vi "Autonomous Independent.vi"   [LabVIEW 2014]
doc: "This VI is called when autonomous begins, and will automatically be terminated when autonomous ends. You can carry out timed or sensor driven robot movement independently without needing to return to the caller."
uses:
  <vilib>/Rock Robotics/WPI/Joystick/WPI_JoystickGetSetRefNum.vi
  <vilib>/Rock Robotics/Network Tables/SD Read Number.vi
  Global 1.vi
panel:
  # "Be sure to right-click and choose Data Operations>>Make Current Value default if you want to save the array values with the VI"
types:
  T1 = typedef "WPI_JoystickDevRef.ctl" = cluster{"Device":T2}
  T2 = typedef "WPI_JoystickDeviceEnum.ctl" = enum16{"USB 0", "USB 1", "USB 2", "USB 3", "USB 4", "USB 5"}
  T3 = typedef "WPI_EncoderDevRef.ctl" = cluster{"DevStatus":errorcluster, "EncoderIndex":T4, "CounterIndex":T5, "DistancePerCount":dbl, "Decoding Type":T6}
  T4 = typedef "FPGA_EncoderIdx.ctl" = enum8{"Enc 0", "Enc 1", "Enc 2", "Enc 3", "Enc 4", "Enc 5", "Enc 6", "Enc 7", "Invalid"}
  T5 = typedef "FPGA_CounterCtrSystemIndex.ctl" = enum8{"Ctr 0", "Ctr 1", "Ctr 2", "Ctr 3", "Ctr 4", "Ctr 5", "Ctr 6", "Ctr 7", "Invalid"}
  T6 = typedef "WPI_EncoderType.ctl" = enum16{"1x", "2x", "4x"}
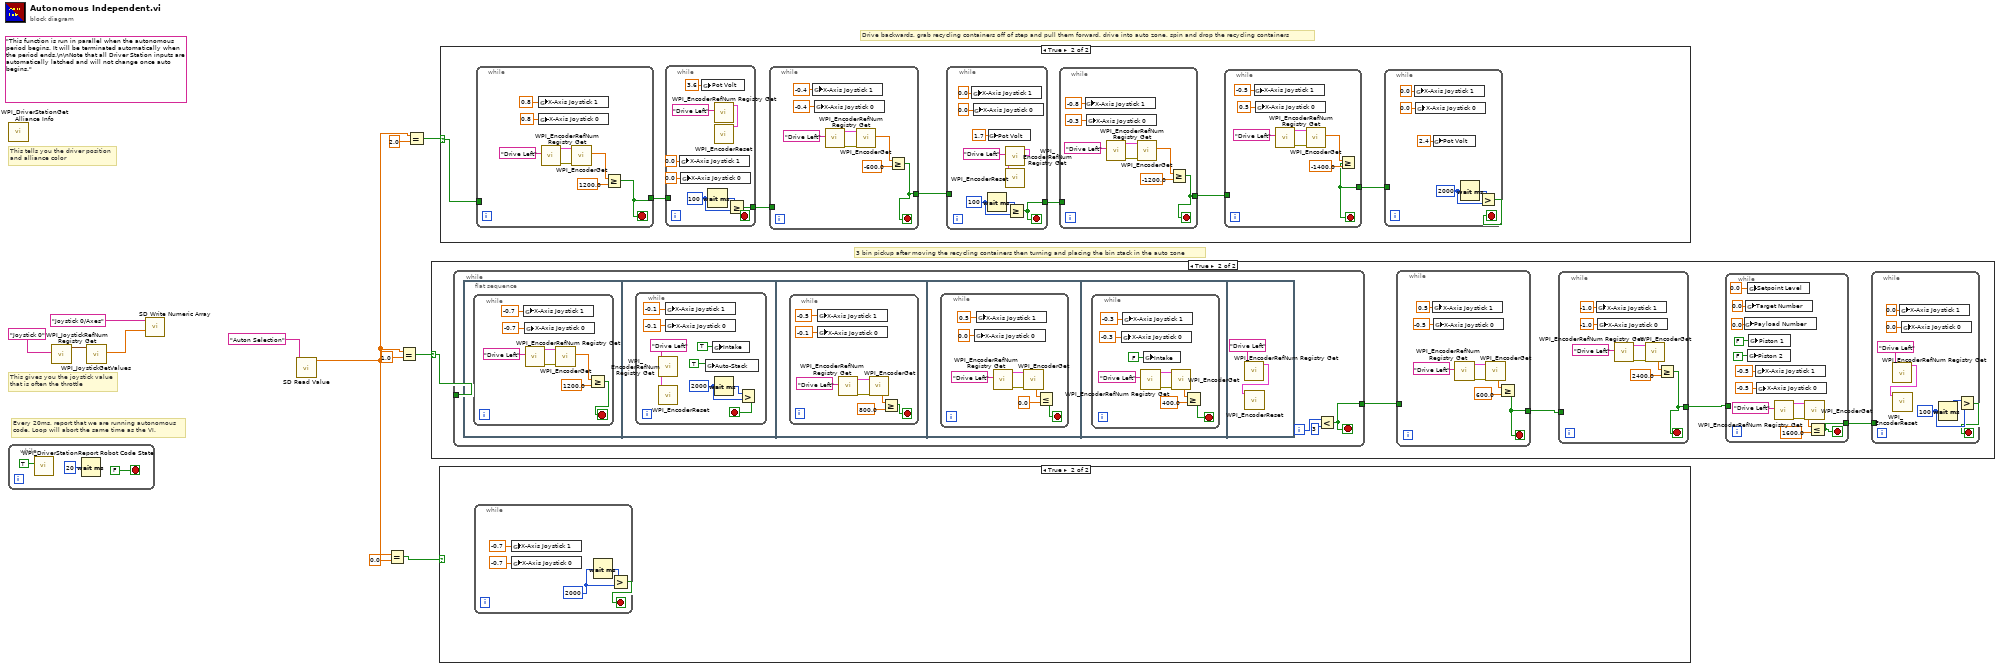
[diagram p0: block diagram]
diagram:
  (unwired) "This function is run in parallel when the autonomous period begins. It will be terminated automatically when the period ends.\n\nNote that all Driver Station inputs are automatically latched and will not change once auto begins."
  # "3 bin pickup after moving the recycling containers then turning and placing the bin stack in the auto zone"
  # "Drive backwards, grab recycling containers off of step and pull them forward, drive into auto zone, spin and drop the recycling containers"
  # "Every 20ms, report that we are running autonomous\ncode. Loop will abort the same time as the VI."
  # "This gives you the joystick value\nthat is often the throttle"
  # "This tells you the driver position\nand alliance color"
  n1 = while {
    stop <- FALSE stop-if-true
    n2 = call <vilib>:"WPI_DriverStationReport Robot Code State.vi"("Autonomous"=TRUE) -> ()  [unwired: 10 in, 1 out]
    n3 = Wait (ms)(milliseconds to wait=u32 20) -> ()  [unwired: 1 out]
  }
  n4 = call <vilib>:"WPI_DriverStationGet Alliance Info.vi"() -> ()  [unwired: 12 out]
  n5 = call <vilib>:"WPI_JoystickRefNum Registry Get.vi"("refnum name"="Joystick 0") -> ("JoystickDevRef"=w11:T1)  [unwired: 1 in, 9 out]
  n6 = call <vilib>:"WPI_JoystickGetValues.vi"("JoystickDevRef"=w11) -> ("Axes"=w9:dbl[])  [unwired: 6 in, 4 out]
  n7 = call <vilib>:"SD Write Numeric Array.vi"("Numeric Array"=w9, "Name"="Joystick 0/Axes") -> ()  [unwired: 8 in, 2 out]
  n8 = call-poly <vilib>:"SD Read Value.vi"("Name"="Auton Selection") -> ("Numeric"=w2:dbl)  [unwired: 8 in, 2 out]
  n9 = Equal?(x=w2, y=0.0) -> (x = y?=w6:bool)
  n10 = Equal?(x=w2, y=1.0) -> (x = y?=w4:bool)
  n11 = Equal?(x=w2, y=2.0) -> (x = y?=w1:bool)
  n12 = case shown="True" w4 {
    selector: w4 -> [_ w20]
    frame False {
    }
    frame True {
      n13 = while {
        tunnel: w20 -> [_]
        tunnel: [w57] -> w19
        i -> [w59]
        stop <- w57 stop-if-true
        n14 = flat-sequence {
          frame #0 {
            n15 = while {
              stop <- w60 stop-if-true
              n16 = global write "Global 1.vi" "X-Axis Joystick 1"(-0.7 ("X-Axis Joystick 1")) -> ()
              n17 = global write "Global 1.vi" "X-Axis Joystick 0"(-0.7 ("X-Axis Joystick 0")) -> ()
              n18 = call <vilib>:"WPI_EncoderRefNum Registry Get.vi"("refnum name"="Drive Left") -> ("error out"=w65:errorcluster, "EncoderDevRef"=w63:T3)  [unwired: 9 in]
              n19 = call <vilib>:"WPI_EncoderGet.vi"("error in (no error)"=w65, "EncoderDevRef"=w63) -> ("Distance"=w62:dbl)  [unwired: 4 in, 5 out]
              n20 = Greater Or Equal?(x=w62, y=1200.0) -> (x >= y?=w60:bool)
            }
          }
          frame #1 {
            n21 = while {
              stop <- w70 stop-if-true
              w71 = u32 2000 ("milliseconds to wait")
              n22 = call <vilib>:"WPI_EncoderRefNum Registry Get.vi"("refnum name"="Drive Left") -> ("EncoderDevRef"=w68:T3)  [unwired: 9 in, 1 out]
              n23 = call <vilib>:"WPI_EncoderReset.vi"("EncoderDevRef"=w68) -> ()  [unwired: 9 in, 2 out]
              n24 = global write "Global 1.vi" "X-Axis Joystick 1"(-0.1 ("X-Axis Joystick 1")) -> ()
              n25 = global write "Global 1.vi" "X-Axis Joystick 0"(-0.1 ("X-Axis Joystick 0")) -> ()
              n26 = global write "Global 1.vi" "Auto-Stack"(TRUE ("Intake")) -> ()
              n27 = global write "Global 1.vi" "Intake"(TRUE ("Intake")) -> ()
              n28 = Wait (ms)(milliseconds to wait=w71) -> (millisecond timer value=w72:u32)
              n29 = Greater?(x=w72, y=w71) -> (0:w70:bool)
            }
          }
          frame #2 {
            n30 = while {
              stop <- w77 stop-if-true
              n31 = global write "Global 1.vi" "X-Axis Joystick 1"(-0.5 ("X-Axis Joystick 1")) -> ()
              n32 = global write "Global 1.vi" "X-Axis Joystick 0"(-0.1 ("X-Axis Joystick 0")) -> ()
              n33 = call <vilib>:"WPI_EncoderRefNum Registry Get.vi"("refnum name"="Drive Left") -> ("error out"=w82:errorcluster, "EncoderDevRef"=w80:T3)  [unwired: 9 in]
              n34 = call <vilib>:"WPI_EncoderGet.vi"("error in (no error)"=w82, "EncoderDevRef"=w80) -> ("Distance"=w79:dbl)  [unwired: 4 in, 5 out]
              n35 = Greater Or Equal?(x=w79, y=800.0) -> (x >= y?=w77:bool)
            }
          }
          frame #3 {
            n36 = while {
              stop <- w85 stop-if-true
              n37 = global write "Global 1.vi" "X-Axis Joystick 0"(0.0 ("X-Axis Joystick 0")) -> ()
              n38 = global write "Global 1.vi" "X-Axis Joystick 1"(0.5 ("X-Axis Joystick 1")) -> ()
              n39 = call <vilib>:"WPI_EncoderRefNum Registry Get.vi"("refnum name"="Drive Left") -> ("error out"=w90:errorcluster, "EncoderDevRef"=w88:T3)  [unwired: 9 in]
              n40 = call <vilib>:"WPI_EncoderGet.vi"("error in (no error)"=w90, "EncoderDevRef"=w88) -> ("Distance"=w87:dbl)  [unwired: 4 in, 5 out]
              n41 = Less Or Equal?(x=w87, y=0.0) -> (x <= y?=w85:bool)
            }
          }
          frame #4 {
            n42 = while {
              stop <- w94 stop-if-true
              n43 = global write "Global 1.vi" "X-Axis Joystick 0"(-0.3 ("X-Axis Joystick 0")) -> ()
              n44 = global write "Global 1.vi" "X-Axis Joystick 1"(-0.3 ("X-Axis Joystick 1")) -> ()
              n45 = call <vilib>:"WPI_EncoderRefNum Registry Get.vi"("refnum name"="Drive Left") -> ("error out"=w99:errorcluster, "EncoderDevRef"=w97:T3)  [unwired: 9 in]
              n46 = global write "Global 1.vi" "Intake"(FALSE ("Intake")) -> ()
              n47 = call <vilib>:"WPI_EncoderGet.vi"("error in (no error)"=w99, "EncoderDevRef"=w97) -> ("Distance"=w96:dbl)  [unwired: 4 in, 5 out]
              n48 = Greater Or Equal?(x=w96, y=400.0) -> (x >= y?=w94:bool)
            }
          }
          frame #5 {
            n49 = call <vilib>:"WPI_EncoderRefNum Registry Get.vi"("refnum name"="Drive Left") -> ("EncoderDevRef"=w102:T3)  [unwired: 9 in, 1 out]
            n50 = call <vilib>:"WPI_EncoderReset.vi"("EncoderDevRef"=w102) -> ()  [unwired: 9 in, 2 out]
          }
        }
        n51 = Less?(x=w59, y=3) -> (x < y?=w57:bool)
      }
      n52 = while {
        tunnel: w19 -> [_]
        tunnel: [w49] -> w18
        stop <- w49 stop-if-true
        n53 = global write "Global 1.vi" "X-Axis Joystick 1"(0.5 ("X-Axis Joystick 1")) -> ()
        n54 = global write "Global 1.vi" "X-Axis Joystick 0"(-0.5 ("X-Axis Joystick 0")) -> ()
        n55 = call <vilib>:"WPI_EncoderRefNum Registry Get.vi"("refnum name"="Drive Left") -> ("error out"=w54:errorcluster, "EncoderDevRef"=w52:T3)  [unwired: 9 in]
        n56 = call <vilib>:"WPI_EncoderGet.vi"("error in (no error)"=w54, "EncoderDevRef"=w52) -> ("Distance"=w51:dbl)  [unwired: 4 in, 5 out]
        n57 = Greater Or Equal?(x=w51, y=600.0) -> (x >= y?=w49:bool)
      }
      n58 = while {
        tunnel: w18 -> [_]
        tunnel: [w41] -> w17
        stop <- w41 stop-if-true
        n59 = global write "Global 1.vi" "X-Axis Joystick 1"(-1.0 ("X-Axis Joystick 1")) -> ()
        n60 = global write "Global 1.vi" "X-Axis Joystick 0"(-1.0 ("X-Axis Joystick 0")) -> ()
        n61 = call <vilib>:"WPI_EncoderRefNum Registry Get.vi"("refnum name"="Drive Left") -> ("error out"=w46:errorcluster, "EncoderDevRef"=w44:T3)  [unwired: 9 in]
        n62 = call <vilib>:"WPI_EncoderGet.vi"("error in (no error)"=w46, "EncoderDevRef"=w44) -> ("Distance"=w43:dbl)  [unwired: 4 in, 5 out]
        n63 = Greater Or Equal?(x=w43, y=2400.0) -> (x >= y?=w41:bool)
      }
      n64 = while {
        tunnel: w17 -> [_]
        tunnel: [w28] -> w16
        stop <- w28 stop-if-true
        n65 = global write "Global 1.vi" "Payload Number"(0.0 ("Setpoint Level")) -> ()
        n66 = global write "Global 1.vi" "Target Number"(0.0 ("Setpoint Level")) -> ()
        n67 = global write "Global 1.vi" "Setpoint Level"(0.0 ("Setpoint Level")) -> ()
        n68 = global write "Global 1.vi" "Piston 2"(FALSE ("Piston 1")) -> ()
        n69 = global write "Global 1.vi" "Piston 1"(FALSE ("Piston 1")) -> ()
        n70 = global write "Global 1.vi" "X-Axis Joystick 1"(-0.5 ("X-Axis Joystick 1")) -> ()
        n71 = global write "Global 1.vi" "X-Axis Joystick 0"(-0.5 ("X-Axis Joystick 0")) -> ()
        n72 = call <vilib>:"WPI_EncoderRefNum Registry Get.vi"("refnum name"="Drive Left") -> ("error out"=w33:errorcluster, "EncoderDevRef"=w31:T3)  [unwired: 9 in]
        n73 = call <vilib>:"WPI_EncoderGet.vi"("error in (no error)"=w33, "EncoderDevRef"=w31) -> ("Distance"=w30:dbl)  [unwired: 4 in, 5 out]
        n74 = Less Or Equal?(x=w30, y=1600.0) -> (x <= y?=w28:bool)
      }
      n75 = while {
        tunnel: w16 -> [_]
        stop <- w21 stop-if-true
        w22 = u32 100 ("milliseconds to wait")
        n76 = call <vilib>:"WPI_EncoderRefNum Registry Get.vi"("refnum name"="Drive Left") -> ("EncoderDevRef"=w24:T3)  [unwired: 9 in, 1 out]
        n77 = call <vilib>:"WPI_EncoderReset.vi"("EncoderDevRef"=w24) -> ()  [unwired: 9 in, 2 out]
        n78 = global write "Global 1.vi" "X-Axis Joystick 1"(0.0 ("X-Axis Joystick 1")) -> ()
        n79 = global write "Global 1.vi" "X-Axis Joystick 0"(0.0 ("X-Axis Joystick 0")) -> ()
        n80 = Wait (ms)(milliseconds to wait=w22) -> (millisecond timer value=w23:u32)
        n81 = Greater?(x=w23, y=w22) -> (0:w21:bool)
      }
    }
  }
  n82 = case shown="True" w6 {
    frame False {
    }
    frame True {
      n83 = while {
        stop <- w104 stop-if-true
        w105 = u32 2000 ("milliseconds to wait")
        n84 = global write "Global 1.vi" "X-Axis Joystick 1"(-0.7 ("X-Axis Joystick 1")) -> ()
        n85 = global write "Global 1.vi" "X-Axis Joystick 0"(-0.7 ("X-Axis Joystick 0")) -> ()
        n86 = Wait (ms)(milliseconds to wait=w105) -> (millisecond timer value=w106:u32)
        n87 = Greater?(x=w106, y=w105) -> (0:w104:bool)
      }
    }
  }
  n88 = case shown="True" w1 {
    selector: w1 -> [_ w115]
    frame False {
    }
    frame True {
      n89 = while {
        tunnel: w115 -> [_]
        tunnel: [w162] -> w114
        stop <- w162 stop-if-true
        n90 = global write "Global 1.vi" "X-Axis Joystick 1"(0.8 ("X-Axis Joystick 1")) -> ()
        n91 = global write "Global 1.vi" "X-Axis Joystick 0"(0.8 ("X-Axis Joystick 0")) -> ()
        n92 = call <vilib>:"WPI_EncoderRefNum Registry Get.vi"("refnum name"="Drive Left") -> ("error out"=w167:errorcluster, "EncoderDevRef"=w165:T3)  [unwired: 9 in]
        n93 = call <vilib>:"WPI_EncoderGet.vi"("error in (no error)"=w167, "EncoderDevRef"=w165) -> ("Distance"=w164:dbl)  [unwired: 4 in, 5 out]
        n94 = Greater Or Equal?(x=w164, y=1200.0) -> (x >= y?=w162:bool)
      }
      n95 = while {
        tunnel: w114 -> [_]
        tunnel: [w155] -> w113
        stop <- w155 stop-if-true
        w156 = u32 100 ("milliseconds to wait")
        n96 = global write "Global 1.vi" "X-Axis Joystick 1"(0.0 ("X-Axis Joystick 1")) -> ()
        n97 = global write "Global 1.vi" "X-Axis Joystick 0"(0.0 ("X-Axis Joystick 0")) -> ()
        n98 = global write "Global 1.vi" "Pot Volt"(3.6 ("Angle")) -> ()
        n99 = Wait (ms)(milliseconds to wait=w156) -> (millisecond timer value=w157:u32)
        n100 = call <vilib>:"WPI_EncoderRefNum Registry Get.vi"("refnum name"="Drive Left") -> ("EncoderDevRef"=w160:T3)  [unwired: 9 in, 1 out]
        n101 = call <vilib>:"WPI_EncoderReset.vi"("EncoderDevRef"=w160) -> ()  [unwired: 9 in, 2 out]
        n102 = Greater Or Equal?(x=w157, y=w156) -> (x >= y?=w155:bool)
      }
      n103 = while {
        tunnel: w113 -> [_]
        tunnel: [w146] -> w112
        stop <- w146 stop-if-true
        n104 = global write "Global 1.vi" "X-Axis Joystick 1"(-0.4 ("X-Axis Joystick 1")) -> ()
        n105 = global write "Global 1.vi" "X-Axis Joystick 0"(-0.4 ("X-Axis Joystick 0")) -> ()
        n106 = call <vilib>:"WPI_EncoderRefNum Registry Get.vi"("refnum name"="Drive Left") -> ("error out"=w151:errorcluster, "EncoderDevRef"=w149:T3)  [unwired: 9 in]
        n107 = call <vilib>:"WPI_EncoderGet.vi"("error in (no error)"=w151, "EncoderDevRef"=w149) -> ("Distance"=w148:dbl)  [unwired: 4 in, 5 out]
        n108 = Greater Or Equal?(x=w148, y=-600.0) -> (x >= y?=w146:bool)
      }
      n109 = while {
        tunnel: w112 -> [_]
        tunnel: [w138] -> w111
        stop <- w138 stop-if-true
        w139 = u32 100 ("milliseconds to wait")
        n110 = global write "Global 1.vi" "X-Axis Joystick 1"(0.0 ("X-Axis Joystick 1")) -> ()
        n111 = global write "Global 1.vi" "X-Axis Joystick 0"(0.0 ("X-Axis Joystick 0")) -> ()
        n112 = Wait (ms)(milliseconds to wait=w139) -> (millisecond timer value=w140:u32)
        n113 = global write "Global 1.vi" "Pot Volt"(1.7 ("Angle")) -> ()
        n114 = call <vilib>:"WPI_EncoderRefNum Registry Get.vi"("refnum name"="Drive Left") -> ("EncoderDevRef"=w141:T3)  [unwired: 9 in, 1 out]
        n115 = call <vilib>:"WPI_EncoderReset.vi"("EncoderDevRef"=w141) -> ()  [unwired: 9 in, 2 out]
        n116 = Greater Or Equal?(x=w140, y=w139) -> (x >= y?=w138:bool)
      }
      n117 = while {
        tunnel: w111 -> [_]
        tunnel: [w130] -> w110
        stop <- w130 stop-if-true
        n118 = global write "Global 1.vi" "X-Axis Joystick 1"(-0.8 ("X-Axis Joystick 1")) -> ()
        n119 = global write "Global 1.vi" "X-Axis Joystick 0"(-0.3 ("X-Axis Joystick 0")) -> ()
        n120 = call <vilib>:"WPI_EncoderRefNum Registry Get.vi"("refnum name"="Drive Left") -> ("error out"=w135:errorcluster, "EncoderDevRef"=w133:T3)  [unwired: 9 in]
        n121 = call <vilib>:"WPI_EncoderGet.vi"("error in (no error)"=w135, "EncoderDevRef"=w133) -> ("Distance"=w132:dbl)  [unwired: 4 in, 5 out]
        n122 = Greater Or Equal?(x=w132, y=-1200.0) -> (x >= y?=w130:bool)
      }
      n123 = while {
        tunnel: w110 -> [_]
        tunnel: [w122] -> w109
        stop <- w122 stop-if-true
        n124 = global write "Global 1.vi" "X-Axis Joystick 1"(-0.5 ("X-Axis Joystick 1")) -> ()
        n125 = global write "Global 1.vi" "X-Axis Joystick 0"(0.5 ("X-Axis Joystick 0")) -> ()
        n126 = call <vilib>:"WPI_EncoderRefNum Registry Get.vi"("refnum name"="Drive Left") -> ("error out"=w127:errorcluster, "EncoderDevRef"=w125:T3)  [unwired: 9 in]
        n127 = call <vilib>:"WPI_EncoderGet.vi"("error in (no error)"=w127, "EncoderDevRef"=w125) -> ("Distance"=w124:dbl)  [unwired: 4 in, 5 out]
        n128 = Greater Or Equal?(x=w124, y=-1400.0) -> (x >= y?=w122:bool)
      }
      n129 = while {
        tunnel: w109 -> [_]
        stop <- w116 stop-if-true
        w117 = u32 2000 ("milliseconds to wait")
        n130 = global write "Global 1.vi" "X-Axis Joystick 1"(0.0 ("X-Axis Joystick 1")) -> ()
        n131 = global write "Global 1.vi" "X-Axis Joystick 0"(0.0 ("X-Axis Joystick 0")) -> ()
        n132 = global write "Global 1.vi" "Pot Volt"(2.4 ("Angle")) -> ()
        n133 = Wait (ms)(milliseconds to wait=w117) -> (millisecond timer value=w118:u32)
        n134 = Greater?(x=w118, y=w117) -> (0:w116:bool)
      }
    }
  }
